vi "EnterButtonPress.vi"(8 "error in (no error)":errorcluster, 11 "View in":refnum<class "View.lvclass">) -> (0 "error out":errorcluster, 2 "endgame?":bool, 3 "View out":refnum<class "View.lvclass">)   [LabVIEW 2024, in "GUI.lvlib" / "View.lvclass"]
uses:
  View.lvclass
  View.lvclass/View.ctl
  <vilib>/Utility/error.llb/Trim Whitespace One-Sided.vi
  Controller/Controller.lvclass
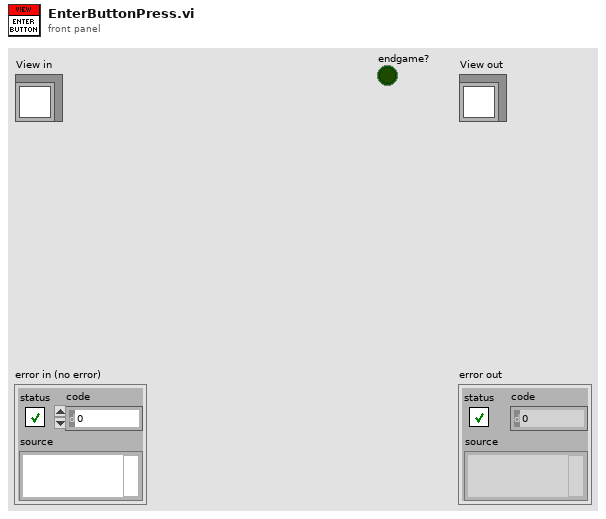
[diagram p1: front panel]
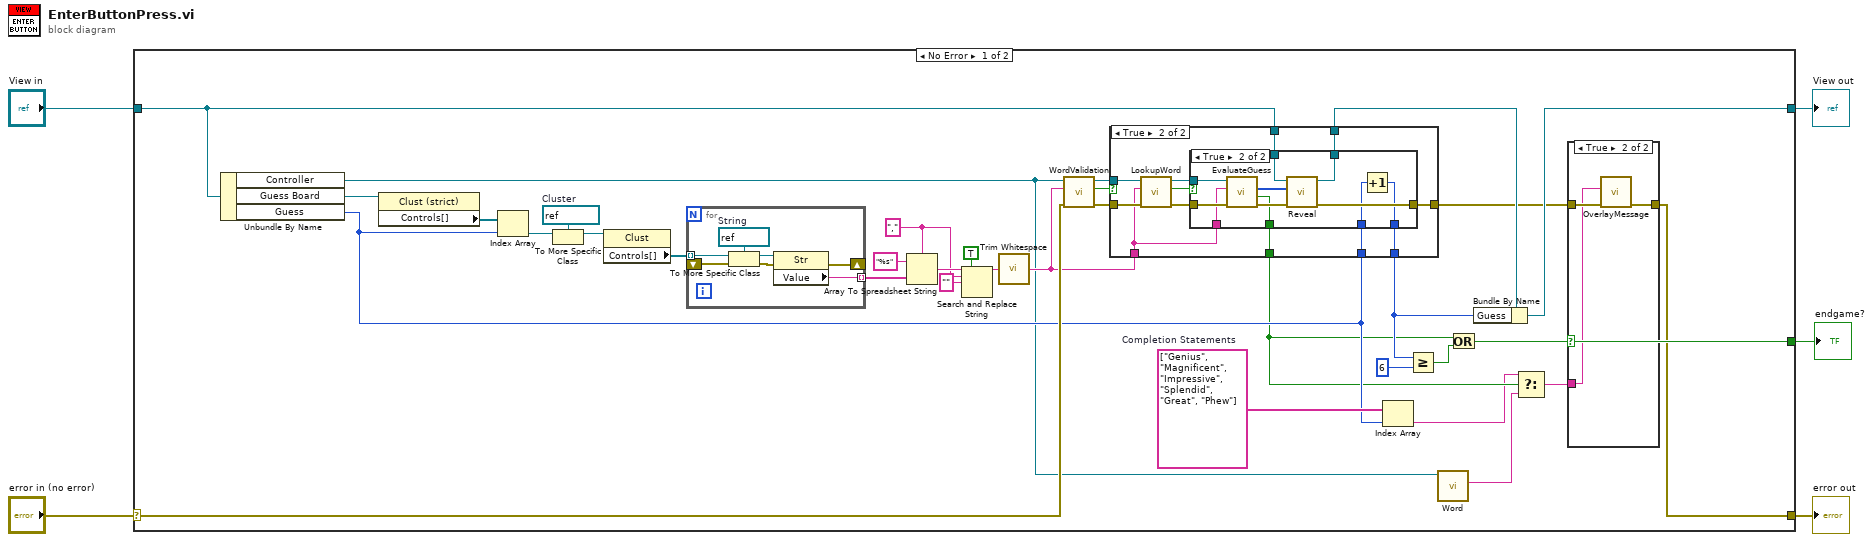
[diagram p0: block diagram]
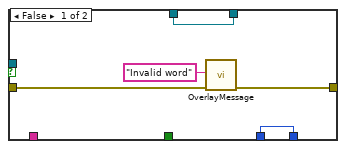
[diagram p3: hidden frame]
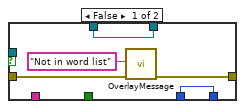
[diagram p4: hidden frame]
diagram:
  n1 = case shown="No Error" "error in (no error)" {
    selector: "error in (no error)" -> [w27 w84]
    tunnel: [w13 w84] -> w4
    tunnel: [w21 w83] -> w2
    tunnel: "View in" -> [w23 w83]
    tunnel: [w17 _] -> w1
    frame No Error {
      w15 = string[] ["Genius", "Magnificent", "Impressive", "Splendid", "Great", "Phew"]  # Completion Statements
      w30 = "," ("delimiter (Tab)")
      w36 = refnum<vi> refnum  # Cluster
      n2 = Unbundle By Name(w23) -> ("Controller"=w6:refnum<class "Controller.lvclass">, "Guess Board"=w39:refnum<vi>, "Guess"=w12:i32)
      n3 = property class="Clust (strict)"(reference=w39) -> ("Controls[]"=w38:refnum<vi>[])  [unwired: 1 in, 2 out]
      n4 = Index Array(array=w38, index=w12) -> (element=w37:refnum<vi>)
      n5 = To More Specific Class(target class=w36, reference=w37) -> (specific class reference=w35:refnum<vi>)  [unwired: 1 in, 1 out]
      n6 = property class="Clust"(reference=w35) -> ("Controls[]"=w34:refnum<vi>[])  [unwired: 1 in, 2 out]
      n7 = for {
        tunnel: w34 -> [w82] mode=indexing
        shift-right: [w77] -> _
        shift-left: _ -> [w80]
        tunnel: [w76] -> w33 mode=indexing
        w81 = refnum<vi> refnum  # String
        n8 = To More Specific Class(target class=w81, reference=w82, error in=w80) -> (specific class reference=w78:refnum<vi>, error out=w79:errorcluster)
        n9 = property class="Str"(reference=w78, error in=w79) -> (error out=w77:errorcluster, "Value"=w76:string)  [unwired: 1 out]
      }
      n10 = Array To Spreadsheet String(delimiter (Tab)=w30, array=w33, 3:"%s" ("format string")) -> (spreadsheet string=w31:string)
      n11 = Search and Replace String(replace all?=TRUE ("replace all? (F)"), input string=w31, search string=w30, replace string="" ("replace string (\"\")")) -> (result string=w24:string)  [unwired: 4 in, 3 out]
      n12 = call <vilib>:"Trim Whitespace.vi"("string"=w24) -> ("trimmed string"=w9:string)  [unwired: 1 in]
      n13 = call "WordValidation.vi"("error in (no error)"=w27, "Word"=w9, "Controller in"=w6) -> ("error out"=w26:errorcluster, "Valid?"=w20:bool, "Controller out"=w25:refnum<class "Controller.lvclass">)  [unwired: 6 in]
      n14 = case shown="True" w20 {
        tunnel: w26 -> [w48 w59]
        tunnel: w25 -> [_ w49]
        tunnel: w9 -> [_ w56]
        tunnel: w23 -> [w46 w55]
        tunnel: [w46 w54] -> w22
        tunnel: [w47 w53] -> w16
        tunnel: [_ w52] -> w11
        tunnel: w12 -> [w44 w51]
        tunnel: [w44 w50] -> w14
        frame False {
          n15 = call "OverlayMessage.vi"("error in (no error)"=w48, "String in"="Invalid word") -> ("error out"=w47:errorcluster)  [unwired: 9 in]
        }
        frame True {
          n16 = call "LookupWord.vi"("error in (no error)"=w59, "Word"=w56) -> ("error out"=w58:errorcluster, "Exists?"=w57:bool)  [unwired: 7 in, 1 out]
          n17 = case shown="True" w57 {
            tunnel: w58 -> [w64 w75]
            tunnel: [w62 w73] -> w53
            tunnel: w56 -> [_ w71]
            tunnel: w55 -> [w61 w70]
            tunnel: [w61 w69] -> w54
            tunnel: [_ w68] -> w52
            tunnel: w51 -> [w60 w67]
            tunnel: [w60 w66] -> w50
            tunnel: w49 -> [_ w65]
            frame False {
              n18 = call "OverlayMessage.vi"("error in (no error)"=w64, "String in"="Not in word list") -> ("error out"=w62:errorcluster)  [unwired: 9 in]
            }
            frame True {
              n19 = call "EvaluateGuess.vi"("error in (no error)"=w75, "Guess"=w71, "Controller in"=w65) -> ("error out"=w74:errorcluster, "correct?"=w68:bool, "Result"=w72:u32[])  [unwired: 5 in, 1 out]
              n20 = call "Reveal.vi"("error in (no error)"=w74, "Result"=w72, "View in"=w70) -> ("error out"=w73:errorcluster, "View out"=w69:refnum<class "View.lvclass">)  [unwired: 7 in]
              n21 = Increment(x=w67) -> (x+1=w66:i32)
            }
          }
        }
      }
      n22 = Index Array(array=w15, index=w12) -> (element=w10:string)
      n23 = Greater Or Equal?(x=w14, y=6) -> (x >= y?=w18:bool)
      n24 = call "Word.vi"("Controller in"=w6) -> ("Word"=w7:string)  [unwired: 8 in, 2 out]
      n25 = Or(x=w11, y=w18) -> (x .or. y?=w17:bool)
      n26 = Bundle By Name(cluster=w22, "Guess"=w14) -> (w21:refnum<class "View.lvclass">)
      n27 = Select(t=w10, s=w11, f=w7) -> (s? t:f=w8:string)
      n28 = case shown="True" w17 {
        tunnel: w16 -> [w40 w43]
        tunnel: w8 -> [_ w42]
        tunnel: [w40 w41] -> w13
        frame False {
        }
        frame True {
          n29 = call "OverlayMessage.vi"("error in (no error)"=w43, "String in"=w42) -> ("error out"=w41:errorcluster)  [unwired: 9 in]
        }
      }
    }
    frame Error {
    }
  }
  "error out" <- w4
  "View out" <- w2
  "endgame?" <- w1
